vi "Log Data.vi"(8 "error in (no error)":cluster{"状态":bool, "代码":i32, "源":string} caption="错误输入（无错误）", 10 "数据队列":refnum<queue>, 11 "记录配置":T1) -> (0 "error out":cluster{"状态":bool, "代码":i32, "源":string} caption="错误输出")   [LabVIEW 2014, in "Logging.lvlib"]
doc: "该VI通过TDMS写入函数将数据写入TDMS文件。"
uses:
  Logging.lvlib
  Logging Configuration.ctl
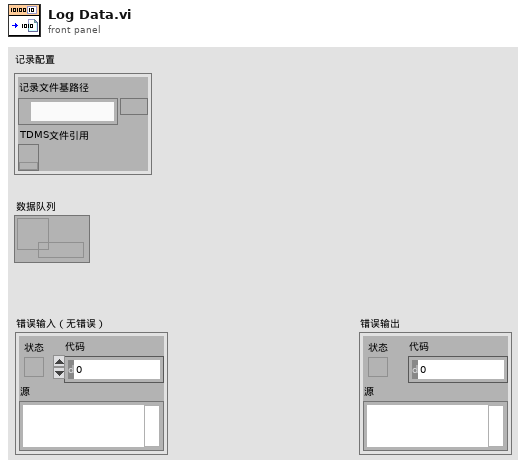
[diagram p1: front panel]
types:
  T1 = typedef "Logging.lvlib/Logging Configuration.ctl" = cluster{"记录文件基路径":path, "TDMS文件引用":refnum<k34>}
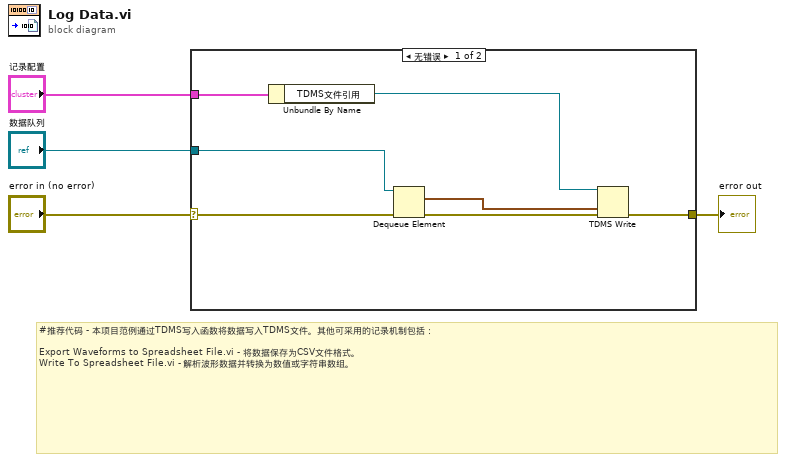
[diagram p0: block diagram]
diagram:
  # "#推荐代码 - 本项目范例通过TDMS写入函数将数据写入TDMS文件。其他可采用的记录机制包括：\n\nExport Waveforms to Spreadsheet File.vi - 将数据保存为CSV文件格式。\nWrite To Spreadsheet File.vi - 解析波形数据并转换为数值或字符串数组。"
  n1 = case shown="无错误" "error in (no error)" {
    selector: "error in (no error)" -> [w9 w12]
    tunnel: "记录配置" -> [w11 _]
    tunnel: "数据队列" -> [w8 _]
    tunnel: [w10 w12] -> w2
    frame No Error {
      n2 = Unbundle By Name(w11) -> ("TDMS文件引用"=w5:refnum<k34>)
      n3 = Dequeue Element(queue=w8, error in (no error)=w9) -> (element=w6:waveform(dbl)[], error out=w7:errorcluster)  [unwired: 1 in, 2 out]
      n4 = TDMS Write(0:w5, 9:w6, 11:w7) -> (15:w10:errorcluster)  [unwired: 3 in, 3 out]
    }
    frame Error {
    }
  }
  "error out" <- w2
